vi "Get most appropriate Local Name and IP.vi"(0 "reset (F)":bool, 5 "target host":string) -> (8 "best source IP":string)   [LabVIEW 2014, in "AMC.lvlib"]
uses:
  AMC.lvlib
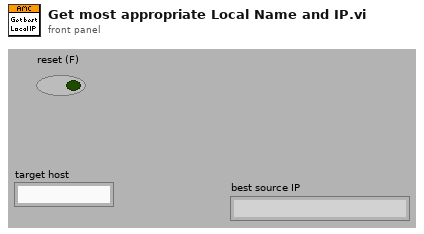
[diagram p1: front panel]
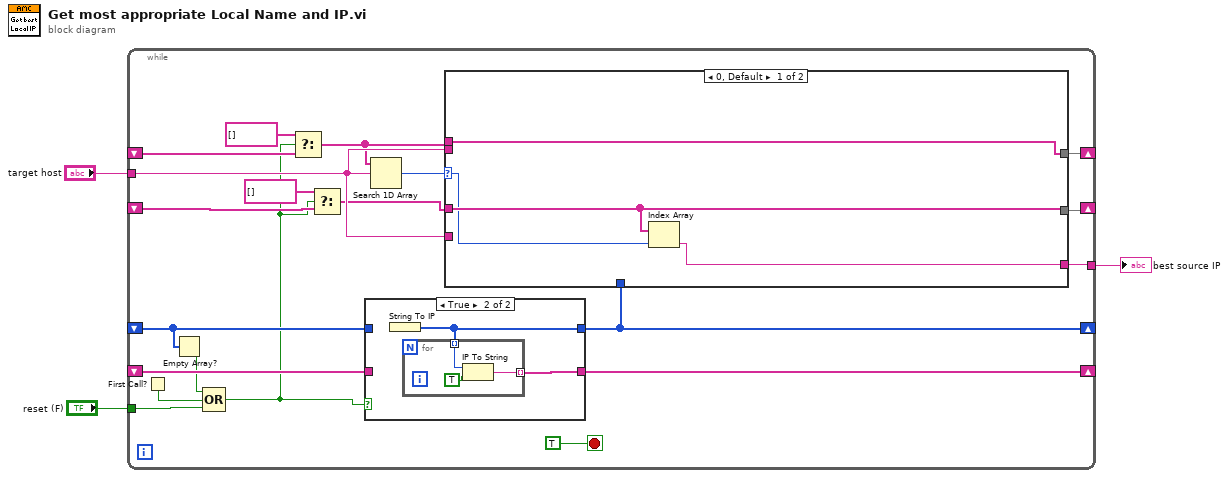
[diagram p0: block diagram]
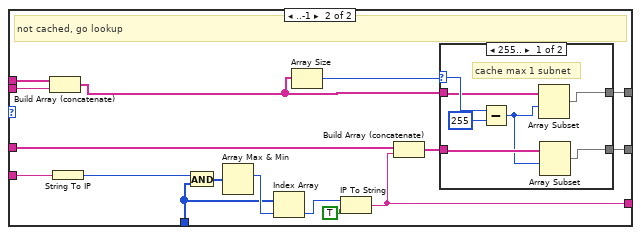
[diagram p2: hidden frame]
diagram:
  n1 = while {
    shift-right: [w12] -> _
    shift-left: _ -> [w18]
    shift-right: [w21] -> _
    shift-left: _ -> [w20]
    tunnel: "reset (F)" -> [w19]
    tunnel: "target host" -> [w11]
    shift-right: [w15] -> _
    shift-left: _ -> [w14]
    shift-right: [w10] -> _
    shift-left: _ -> [w8]
    tunnel: [w5] -> w1
    stop <- TRUE stop-if-true
    n2 = First Call?() -> (First Call?: T/F=w22:bool)
    n3 = Empty Array?(array=w18) -> (empty?=w17:bool)
    n4 = Compound Arithmetic op=OR(w17, w22, w19) -> (w6:bool)
    n5 = Select(t=string[] [], s=w6, f=w14) -> (s? t:f=w4:string[])
    n6 = Select(t=string[] [], s=w6, f=w8) -> (s? t:f=w7:string[])
    n7 = case shown="True" w6 {
      tunnel: [w54 w55] -> w12
      tunnel: [w53 w56] -> w21
      tunnel: w18 -> [w54 _]
      tunnel: w20 -> [w53 _]
      frame False {
      }
      frame True {
        n8 = String To IP() -> (0:w55:u32[])  [unwired: 1 out]
        n9 = for {
          tunnel: [w58] -> w56 mode=indexing
          tunnel: w55 -> [w57] mode=indexing
          n10 = IP To String(1:TRUE ("dot notation? (F)"), 2:w57) -> (0:w58:string)
        }
      }
    }
    n11 = Search 1D Array(1D array=w4, element=w11) -> (index of element=w16:i32)  [unwired: 1 in]
    n12 = case shown="0, Default" w16 {
      selector: w16 -> [w25 _]
      tunnel: w11 -> [_ w43]
      tunnel: [w27 w30] -> w15
      tunnel: w4 -> [w27 w42]
      tunnel: w12 -> [_ w37]
      tunnel: w11 -> [_ w41]
      tunnel: [w26 w28] -> w10
      tunnel: w7 -> [w26 w34]
      tunnel: [w24 w33] -> w5
      frame 0, Default {
        n13 = Index Array(array=w26, index=w25) -> (element=w24:string)
      }
      frame ..-1 {
        # "not cached, go lookup"
        n14 = Build Array (concatenate)(w42, w43) -> (w29:string[])
        n15 = String To IP(1:w41) -> (0:w40:u32)
        n16 = And(x=w40, y=w37) -> (x .and. y?=w39:u32[])
        n17 = Array Max & Min(array=w39) -> (max index (indices)=w38:i32)  [unwired: 3 out]
        n18 = Index Array(array=w37, index=w38) -> (element=w35:u32)
        n19 = Array Size(array=w29) -> (size(s)=w31:i32)
        n20 = IP To String(1:TRUE ("dot notation? (F)"), 2:w35) -> (0:w33:string)
        n21 = Build Array (concatenate)(w34, w33) -> (w32:string[])
        n22 = case shown="255.." w31 {
          selector: w31 -> [w50 _]
          tunnel: w32 -> [w47 w51]
          tunnel: [w44 w52] -> w30
          tunnel: w29 -> [w48 w52]
          tunnel: [w45 w51] -> w28
          frame 255.. {
            # "cache max 1 subnet"
            n23 = Subtract(x=w50, y=255) -> (x-y=w46:i32)
            n24 = Array Subset(array=w48, index=w46) -> (w44:string[])  [unwired: 1 in]
            n25 = Array Subset(array=w47, index=w46) -> (w45:string[])  [unwired: 1 in]
          }
          frame Default {
          }
        }
      }
    }
  }
  "best source IP" <- w1
